vi "ABAPI Dist Recursive Delete Temp.vi"(2 "error in (no error)":errorcluster, 3 "path":path) -> (0 "error out":errorcluster)   [LabVIEW 2020]
panel:
  in  "Skip it":bool
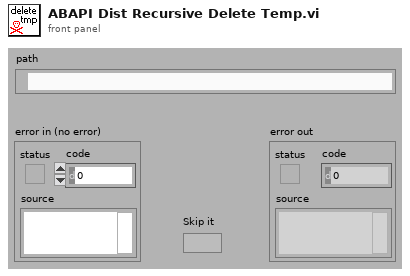
[diagram p1: front panel]
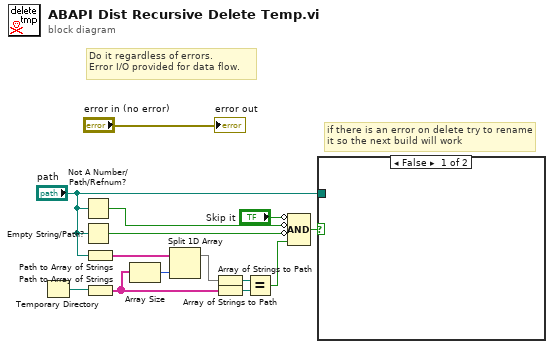
[diagram p0: block diagram]
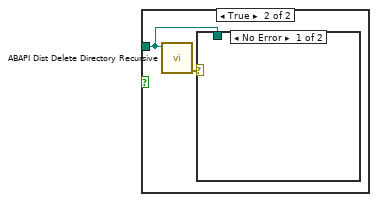
[diagram p2: hidden frame]
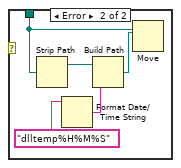
[diagram p3: hidden frame]
diagram:
  # "if there is an error on delete try to rename it so the next build will work"
  # "Do it regardless of errors.\nError I/O provided for data flow."
  n1 = Temporary Directory() -> (w13:path)
  n2 = Not A Number/Path/Refnum?(number/path/refnum="path") -> (NaN/Path/Refnum?=w10:bool)
  n3 = Empty String/Path?(string/path="path") -> (empty?=w9:bool)
  n4 = Path to Array of Strings(0:"path") -> (2:w12:string[])  [unwired: 1 out]
  n5 = Path to Array of Strings(0:w13) -> (2:w4:string[])  [unwired: 1 out]
  n6 = Array Size(array=w4) -> (size(s)=w11:i32)
  n7 = Split 1D Array(array=w12, index=w11) -> (first subarray=w6:string[])  [unwired: 1 out]
  n8 = Array of Strings to Path(0:w6) -> (2:w3:path)  [unwired: 1 in]
  n9 = Array of Strings to Path(0:w4) -> (2:w5:path)  [unwired: 1 in]
  n10 = Equal?(x=w3, y=w5) -> (x = y?=w8:bool)
  n11 = Compound Arithmetic op=AND(invert "Skip it", invert w10, invert w9, w8) -> (w7:bool)
  n12 = case shown="False" w7 {
    tunnel: "path" -> [_ w16]
    frame False {
    }
    frame True {
      n13 = call <vilib>:"ABAPI Dist Delete Directory Recursive.vi"("directory"=w16) -> ("error out"=w15:errorcluster)  [unwired: 10 in]
      n14 = case shown="No Error" w15 {
        tunnel: w16 -> [_ w17]
        frame No Error {
        }
        frame Error {
          n15 = Strip Path(path=w17) -> (stripped path=w20:path)  [unwired: 1 out]
          n16 = Format Date/Time String(time format string (%c)="dlltemp%H%M%S") -> (date/time string=w19:string)  [unwired: 2 in]
          n17 = Build Path(base path=w20, name or relative path=w19) -> (appended path=w21:path)
          n18 = Move(source path=w17, 10:w21) -> ()  [unwired: 3 in, 3 out]
        }
      }
    }
  }
  "error out" <- "error in (no error)"
